vi "FusePose.vi"(0 "LimeLight deltaX":dbl, 1 "Odometry deltaY":dbl, 2 "Odometry deltaX":dbl, 5 "LimeLight deltaY":dbl, 12 "LimeLight Pose Valid":bool) -> (4 "Fused deltaX":dbl, 15 "Fused deltaY":dbl)   [LabVIEW 2019]
doc: "This VI fuses multiple sensing modalities to estimate the robot's current pose."
uses:
  dsdata.vi
  <vilib>/Rock Robotics/WPI/DriverStation/WPI_DriverStationRobotMode2.ctl
panel:
  in  "Max Y Error (in)":dbl=240.0
  in  "Max X Error (in)":dbl=240.0
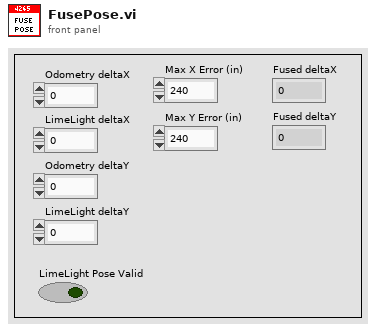
[diagram p1: front panel]
types:
  T1 = typedef "WPI_DriverStationRobotMode2.ctl" = enum16{"Autonomous Disabled", "Autonomous Enabled", "Teleop Disabled", "Teleop Enabled", "Disconnected", "Finish", "Test Disabled", "Test Enabled", "Emergency Stopped"}
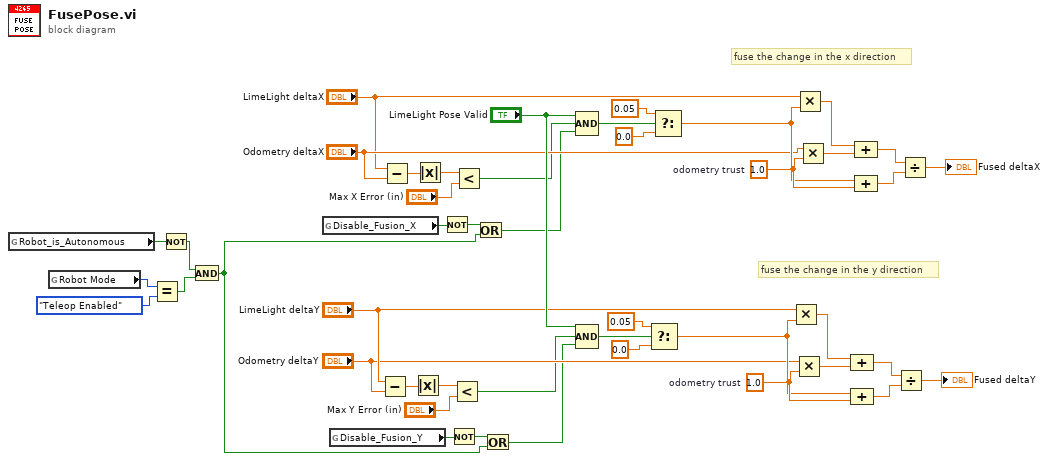
[diagram p0: block diagram]
diagram:
  w33 = 1.0  # odometry trust
  w42 = 1.0  # odometry trust
  # "fuse the change in the y direction"
  # "fuse the change in the x direction"
  n1 = global read "dsdata.vi" "Robot_is_Autonomous"() -> (w6:bool)
  n2 = global read "dsdata.vi" "Robot Mode"() -> (w5:T1)
  n3 = Equal?(x=w5, y=WPI_DriverStationRobotMode2."Teleop Enabled") -> (x = y?=w4:bool)
  n4 = Not(x=w6) -> (.not. x?=w3:bool)
  n5 = And(x=w3, y=w4) -> (x .and. y?=w2:bool)
  n6 = global read "dsdata.vi" "Disable_Fusion_X"() -> (w12:bool)
  n7 = global read "dsdata.vi" "Disable_Fusion_Y"() -> (w9:bool)
  n8 = Subtract(x="LimeLight deltaY", y="Odometry deltaY") -> (x-y=w19:dbl)
  n9 = Subtract(x="LimeLight deltaX", y="Odometry deltaX") -> (x-y=w22:dbl)
  n10 = Absolute Value(x=w19) -> (abs(x)=w18:dbl)
  n11 = Absolute Value(x=w22) -> (abs(x)=w21:dbl)
  n12 = Not(x=w12) -> (.not. x?=w11:bool)
  n13 = Not(x=w9) -> (.not. x?=w8:bool)
  n14 = Less?(x=w18, y="Max Y Error (in)") -> (x < y?=w14:bool)
  n15 = Less?(x=w21, y="Max X Error (in)") -> (x < y?=w13:bool)
  n16 = Or(x=w11, y=w2) -> (x .or. y?=w10:bool)
  n17 = Or(x=w8, y=w2) -> (x .or. y?=w7:bool)
  n18 = Compound Arithmetic op=AND("LimeLight Pose Valid", w13, w10) -> (w27:bool)
  n19 = Compound Arithmetic op=AND("LimeLight Pose Valid", w14, w7) -> (w26:bool)
  n20 = Select(t=0.05, s=w26, f=0.0) -> (s? t:f=w29:dbl)
  n21 = Select(t=0.05, s=w27, f=0.0) -> (s? t:f=w38:dbl)
  n22 = Multiply(x="LimeLight deltaY", y=w29) -> (x*y=w32:dbl)
  n23 = Multiply(x="Odometry deltaY", y=w33) -> (x*y=w34:dbl)
  n24 = Multiply(x="LimeLight deltaX", y=w38) -> (x*y=w41:dbl)
  n25 = Multiply(x="Odometry deltaX", y=w42) -> (x*y=w43:dbl)
  n26 = Compound Arithmetic op=ADD(w32, w34) -> (w35:dbl)
  n27 = Compound Arithmetic op=ADD(w29, w33) -> (w36:dbl)
  n28 = Compound Arithmetic op=ADD(w41, w43) -> (w44:dbl)
  n29 = Compound Arithmetic op=ADD(w38, w42) -> (w45:dbl)
  n30 = Divide(x=w35, y=w36) -> (x/y=→"Fused deltaY":dbl)
  n31 = Divide(x=w44, y=w45) -> (x/y=→"Fused deltaX":dbl)
